vi "save internal files.vi"(8 "error in (no error)":errorcluster, 11 "device_type in":refnum<class "device_type.lvclass">) -> (0 "error out":errorcluster, 3 "device_type out":refnum<class "device_type.lvclass">)   [LabVIEW 2021, in "device_type.lvclass"]
uses:
  device_type.lvclass
  device_type.lvclass/device_type.ctl
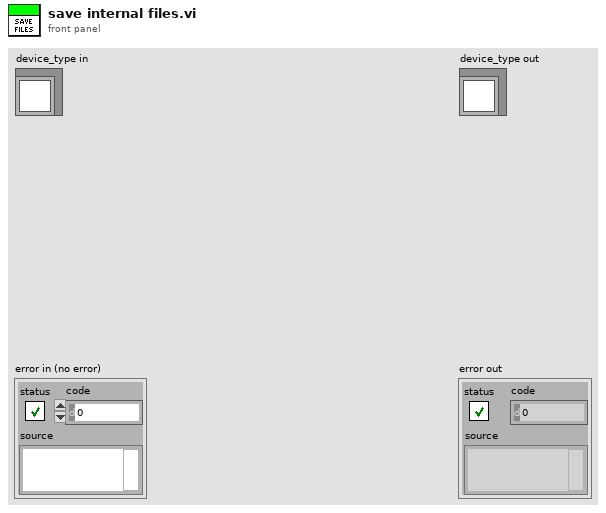
[diagram p1: front panel]
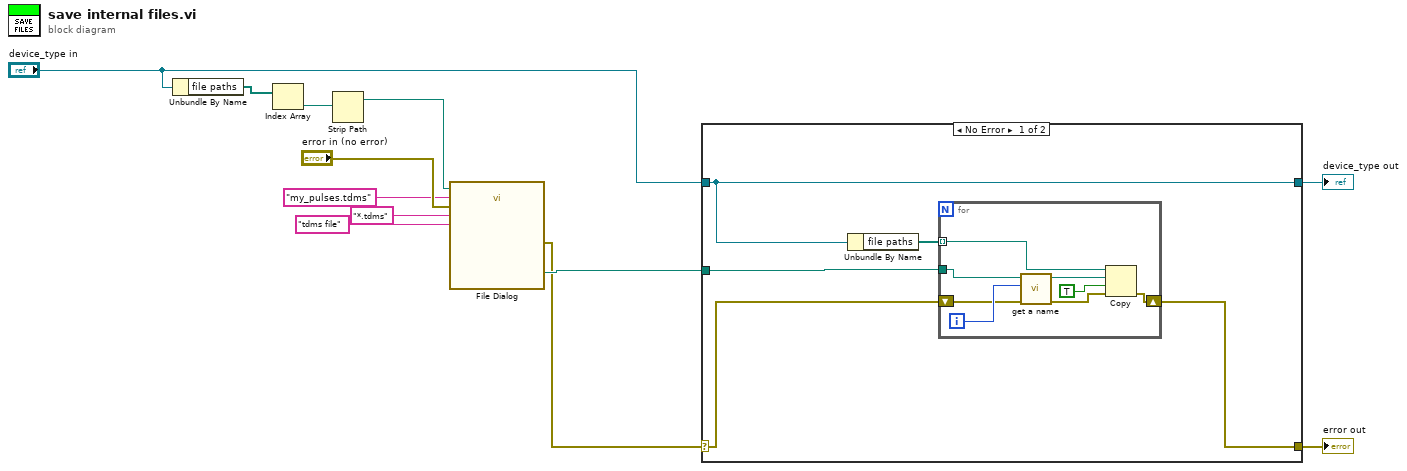
[diagram p0: block diagram]
diagram:
  n1 = Unbundle By Name("device_type in") -> ("file paths"=w3:path[])
  n2 = Index Array(array=w3) -> (element=w2:path)  [unwired: 1 in]
  n3 = Strip Path(path=w2) -> (stripped path=w1:path)  [unwired: 1 out]
  n4 = call "File Dialog"("start path"=w1, "default name"="my_pulses.tdms", "error in"="error in (no error)", "pattern (all files)"="*.tdms", "pattern label"="tdms file") -> ("selected path"=w10:path, "error out"=w7:errorcluster)  [unwired: 7 in, 2 out]
  n5 = case shown="No Error" w7 {
    selector: w7 -> [w14 w27]
    tunnel: [w13 w27] -> w12
    tunnel: [w17 w26] -> w11
    tunnel: "device_type in" -> [w17 w26]
    tunnel: w10 -> [w15 _]
    frame No Error {
      n6 = Unbundle By Name(w17) -> ("file paths"=w16:path[])
      n7 = for {
        tunnel: w16 -> [w25] mode=indexing
        tunnel: w15 -> [w18]
        shift-right: [w20] -> w13
        shift-left: w14 -> [w22]
        i -> [w24]
        n8 = call "get a name.vi"("error constant"=w22, "Numeric"=w24, "Bitfile path"=w18) -> ("error constant 2"=w21:errorcluster, "Path"=w19:path)  [unwired: 7 in]
        n9 = Copy(8:w21, 9:TRUE ("overwrite (F)"), 10:w19, 11:w25) -> (0:w20:errorcluster)  [unwired: 1 in, 2 out]
      }
    }
    frame Error {
    }
  }
  "error out" <- w12
  "device_type out" <- w11
